vi "Temp Array Gen.1.vi"(8 "error in (no error)":errorcluster, 11 "Temperature Control Parameters":T1 {"End Temp" format="%.2f"; "Temp Step" format="%.2f"; "Start Temp" format="%.2f"}) -> (0 "error out":errorcluster)   [LabVIEW 2014]
doc: "Temp Array Gen\n\nCreates an array of temperature given the starting, step, end temperature. This should return an array and the number of temperatures. Takes in consideration inverted limits and steps of zero.\n\nBeverly Abadines\nPHY 350 \nBAP3B"
uses:
  typedefs/temp control params.ctl
panel:
  out "Temp Array 2":dbl[](array[numeric])
  out "N Temps":i32=6
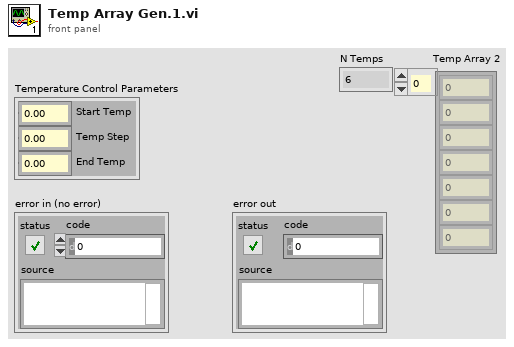
[diagram p1: front panel]
types:
  T1 = typedef "temp control params.ctl" = cluster{"Start Temp":dbl, "Temp Step":dbl, "End Temp":dbl}
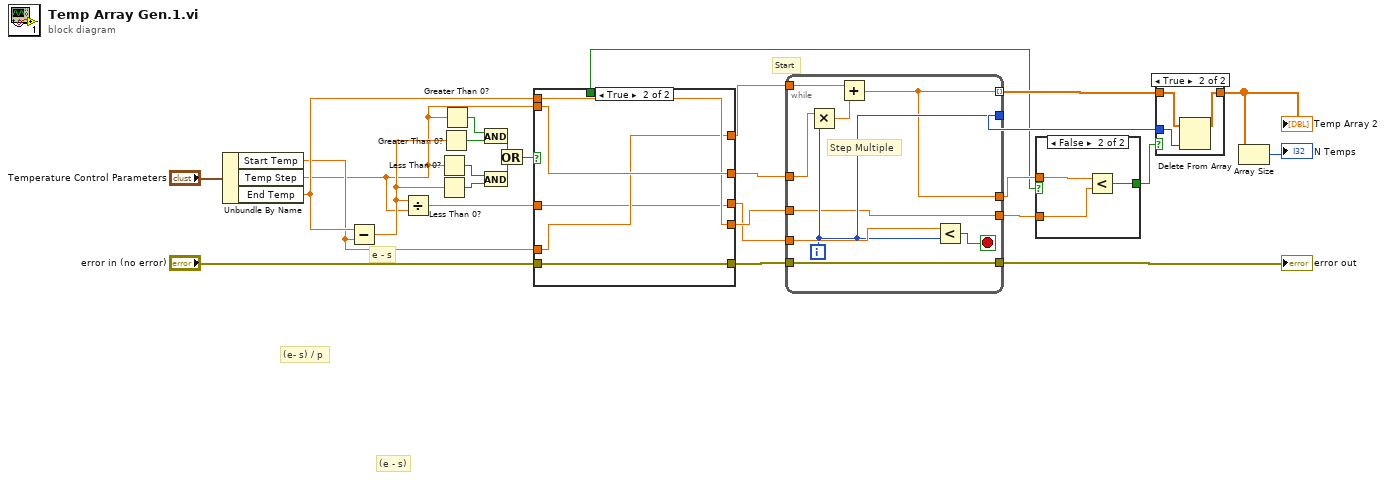
[diagram p0: block diagram]
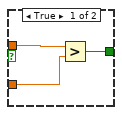
[diagram p2: hidden frame]
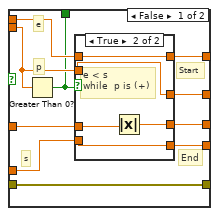
[diagram p3: hidden frame]
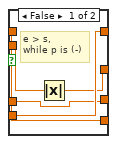
[diagram p4: hidden frame]
diagram:
  # "(e - s)"
  # "(e- s) / p"
  # "e - s"
  # "Start"
  n1 = Unbundle By Name("Temperature Control Parameters") -> ("Start Temp"=w18:dbl, "Temp Step"=w12:dbl, "End Temp"=w20:dbl)
  n2 = Subtract(x=w20, y=w18) -> (x-y=w13:dbl)
  n3 = Divide(x=w13, y=w12) -> (x/y=w6:dbl)
  n4 = Less Than 0?(x=w12) -> (x < 0?=w10:bool)
  n5 = Less Than 0?(x=w13) -> (x < 0?=w11:bool)
  n6 = Greater Than 0?(x=w13) -> (x > 0?=w21:bool)
  n7 = Greater Than 0?(x=w12) -> (x > 0?=w22:bool)
  n8 = And(x=w22, y=w21) -> (x .and. y?=w15:bool)
  n9 = And(x=w10, y=w11) -> (x .and. y?=w9:bool)
  n10 = Or(x=w15, y=w9) -> (x .or. y?=w14:bool)
  n11 = case shown="True" w14 {
    tunnel: w12 -> [w34 w53]
    tunnel: w20 -> [w38 w52]
    tunnel: [w37 w51] -> w19
    tunnel: w18 -> [w36 w51]
    tunnel: [w35 w52] -> w17
    tunnel: [w33 w53] -> w16
    tunnel: "error in (no error)" -> [w32 w50]
    tunnel: [w32 w50] -> w7
    tunnel: w6 -> [w31 w49]
    tunnel: [w30 w49] -> w5
    tunnel: [w29 _] -> w1
    frame False {
      # "p"
      # "e"
      # "s"
      # "End"
      # "Start"
      n12 = Greater Than 0?(x=w34) -> (x > 0?=w29:bool)
      n13 = case shown="True" w29 {
        tunnel: w38 -> [w42 w48]
        tunnel: [w43 w48] -> w37
        tunnel: w36 -> [w43 w47]
        tunnel: [w42 w47] -> w35
        tunnel: w34 -> [w41 w46]
        tunnel: [w40 w46] -> w33
        tunnel: w31 -> [w39 w45]
        tunnel: [w39 w44] -> w30
        frame False {
          # "e > s,\nwhile p is (-)"
          n14 = Absolute Value(x=w41) -> (abs(x)=w40:dbl)
        }
        frame True {
          # "e < s\nwhile  p is (+)"
          n15 = Absolute Value(x=w45) -> (abs(x)=w44:dbl)
        }
      }
    }
    frame True {
    }
  }
  n16 = while {
    tunnel: w19 -> [w60]
    tunnel: w16 -> [w62]
    tunnel: [w55] -> w26 mode=indexing
    tunnel: w5 -> [w59]
    tunnel: [w58] -> w25
    tunnel: w7 -> [w57]
    tunnel: [w57] -> w23
    tunnel: w17 -> [w54]
    tunnel: [w55] -> w4
    tunnel: [w54] -> w3
    i -> [w58]
    stop <- w56 stop-if-true
    # "Step Multiple"
    n17 = Multiply(x=w62, y=w58) -> (x*y=w61:dbl)
    n18 = Add(x=w60, y=w61) -> (x+y=w55:dbl)
    n19 = Less?(x=w59, y=w58) -> (x < y?=w56:bool)
  }
  "error out" <- w23
  n20 = case shown="False" w1 {
    tunnel: w4 -> [w65 w68]
    tunnel: w3 -> [w64 w67]
    tunnel: [w63 w66] -> w2
    frame True {
      n21 = Greater?(x=w65, y=w64) -> (0:w63:bool)
    }
    frame False {
      n22 = Less?(x=w68, y=w67) -> (x < y?=w66:bool)
    }
  }
  n23 = case shown="True" w2 {
    tunnel: w26 -> [w69 w72]
    tunnel: [w69 w71] -> w24
    tunnel: w25 -> [_ w70]
    frame False {
    }
    frame True {
      n24 = Delete From Array(array=w72, index=w70) -> (array with subset deleted=w71:dbl[])  [unwired: 1 in, 1 out]
    }
  }
  "Temp Array 2" <- w24
  n25 = Array Size(array=w24) -> (size(s)=→"N Temps":i32)
